vi "Get syringe map.vi"() -> (0 "Offset map (2D 1 row)":dbl[][](array[numeric]), 1 "Syringe map":dbl[](array[numeric]))   [LabVIEW 2021]
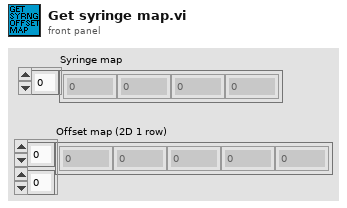
[diagram p1: front panel]
types:
  T1 = typedef "File Paths.ctl" = cluster{"Glue Pattern Folder":path, "Carrier Tray Folder":path, "Pick Up Tool Fixture Folder":path, "Components Folder":path, "Bellows Tool Offset.txt":path, "Pick Up Tool Offset.txt":path, "Dispense Tip Offset.txt":path, "Log Files":path, "Gantry Assembly Map.txt":path, "Syringe and offset map.txt":path, "Controllers Folder":path, "Local dbase config":path}
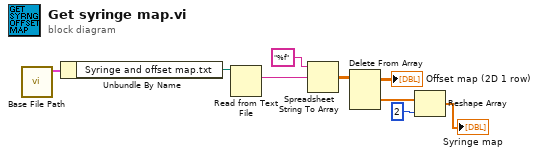
[diagram p0: block diagram]
diagram:
  n1 = call "Base File Path.vi"() -> ("Paths Out"=w2:T1)  [unwired: 11 in]
  n2 = Unbundle By Name(w2) -> ("Syringe and offset map.txt"=w1:path)
  n3 = Read from Text File(file (use dialog)=w1) -> (text=w9:string)  [unwired: 3 in, 3 out]
  n4 = Spreadsheet String To Array(format string="%f", spreadsheet string=w9) -> (array=w7:dbl[][])  [unwired: 2 in]
  n5 = Delete From Array(array=w7) -> (deleted portion=w4:dbl[], array with subset deleted=→"Offset map (2D 1 row)":dbl[][])  [unwired: 3 in]
  n6 = Reshape Array(w4, 2) -> (→"Syringe map":dbl[])
